vi "Change Message Visibility (Batch).vi"(8 "error in (no error)":errorcluster, 9 "Visibility Timeouts":i32[](array[numeric]), 10 "Receipt Handles":string[](array[string]), 11 "SQS in":refnum<class "NI_AWS_SQS.lvclass">) -> (0 "error out":errorcluster, 3 "SQS out":refnum<class "NI_AWS_SQS.lvclass">)   [LabVIEW 2015, in "NI_AWS_SQS.lvclass"]
uses:
  NI_AWS_SQS.lvclass
  Core/Name Value Pair.ctl
  Core/Request Options.ctl
  NI_AWS_SQS.lvclass/NI_AWS_SQS.ctl
  Read Account Number.vi
  Read Name.vi
  Core/NI_AWS_Core.lvclass
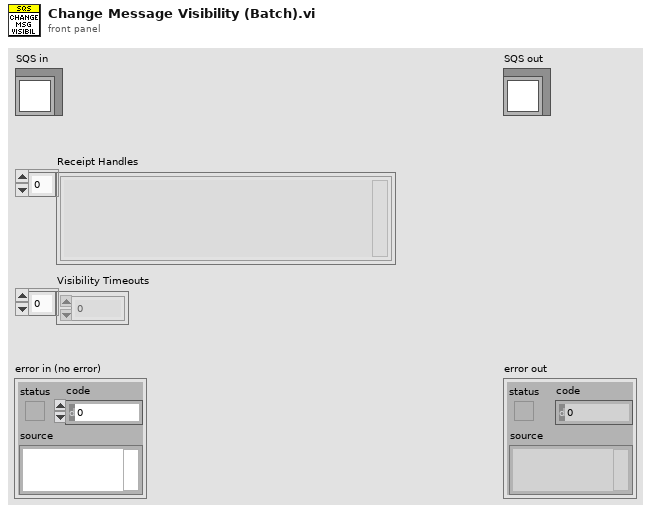
[diagram p1: front panel]
types:
  T1 = typedef "NI_AWS_Core.lvclass/Request Options.ctl" = cluster{"request headers":T2[], "request parameters":T2[], "request body":string}
  T2 = typedef "NI_AWS_Core.lvclass/Name Value Pair.ctl" = cluster{"name":string, "value":string}
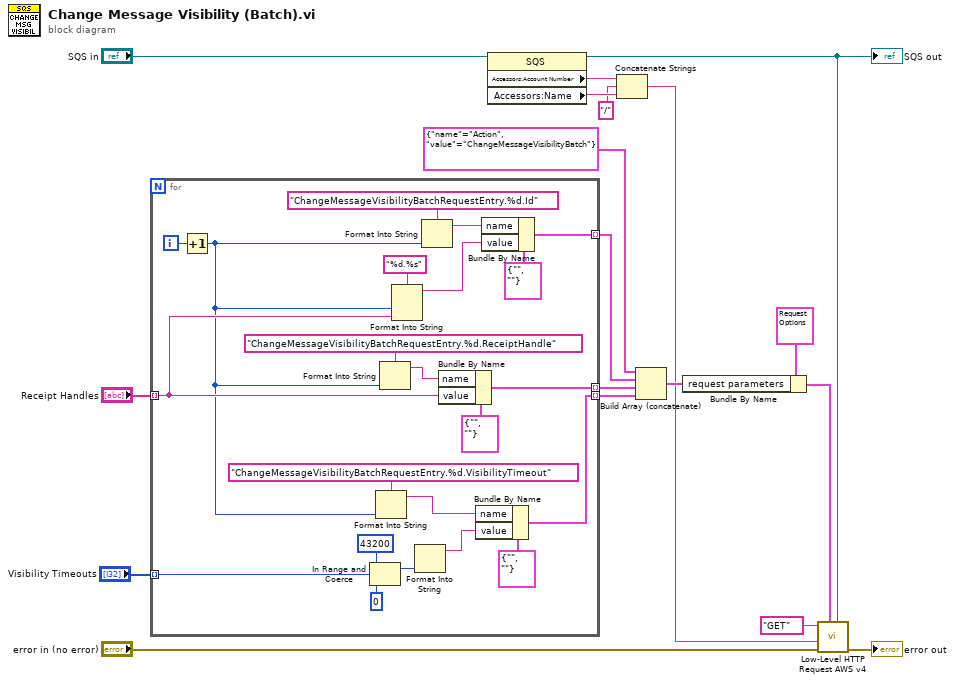
[diagram p0: block diagram]
diagram:
  n1 = for {
    tunnel: [w39] -> w6 mode=indexing
    tunnel: [w37] -> w5 mode=indexing
    tunnel: "Receipt Handles" -> [w22] mode=indexing
    tunnel: "Visibility Timeouts" -> [w32] mode=indexing
    tunnel: [w29] -> w1 mode=indexing
    i -> [w30]
    n2 = Increment(x=w30) -> (x+1=w19:i32)
    n3 = In Range and Coerce(upper limit=43200, x=w32, lower limit=0) -> (coerced(x)=w34:i32)  [unwired: 1 out]
    n4 = Format Into String(format string="ChangeMessageVisibilityBatchRequestEntry.%d.VisibilityTimeout" ("name"), w19) -> (resulting string=w20:string)  [unwired: 2 in, 1 out]
    n5 = Format Into String(format string="ChangeMessageVisibilityBatchRequestEntry.%d.ReceiptHandle" ("name"), w19) -> (resulting string=w23:string)  [unwired: 2 in, 1 out]
    n6 = Format Into String(format string="%d.%s", w19, w22) -> (resulting string=w25:string)  [unwired: 2 in, 1 out]
    n7 = Format Into String(w34) -> (resulting string=w33:string)  [unwired: 3 in, 1 out]
    n8 = Format Into String(format string="ChangeMessageVisibilityBatchRequestEntry.%d.Id" ("name"), w19) -> (resulting string=w28:string)  [unwired: 2 in, 1 out]
    n9 = Bundle By Name(cluster=T2 {"name"="", "value"=""} ("element"), "name"=w23, "value"=w22) -> (w39:T2)
    n10 = Bundle By Name(cluster=T2 {"name"="", "value"=""} ("element"), "name"=w20, "value"=w33) -> (w37:T2)
    n11 = Bundle By Name(cluster=T2 {"name"="", "value"=""} ("element"), "name"=w28, "value"=w25) -> (w29:T2)
  }
  n12 = property class="SQS"(reference="SQS in") -> (reference out=w11:refnum<class "NI_AWS_SQS.lvclass">, "Accessors:Account Number"=w10:string, "Accessors:Name"=w9:string)  [unwired: 1 in, 1 out]
  "SQS out" <- w11
  n13 = Concatenate Strings(w10, "/", w9) -> (w7:string)
  n14 = Build Array (concatenate)(T2 {"name"="Action", "value"="ChangeMessageVisibilityBatch"} ("Cluster"), w1, w6, w5) -> (w12:T2[])
  n15 = Bundle By Name(cluster=T1 {"request headers"=[], "request parameters"=[{"name"="Action", "value"="ListQueues"}], "request body"=""} ("Request Options"), "request parameters"=w12) -> (w13:T1)
  n16 = call "Low-Level HTTP Request AWS v4.vi"("AWS Core"=w11, "Request Options"=w13, "error in (no error)"="error in (no error)", "URL Suffix"=w7, "HTTP-Verb"="GET") -> ("error out"=→"error out":errorcluster)  [unwired: 4 in, 2 out]
